vi "Close File.vi"(8 "error in (no error)":errorcluster, 11 "Parameter INI File in":refnum<class "Parameter INI File.lvclass">) -> (0 "error out":errorcluster, 3 "Parameter INI File out":refnum<class "Parameter INI File.lvclass">)   [LabVIEW 2016, in "CD Parameter Manager API.lvlib" / "Parameter INI File.lvclass"]
uses:
  Parameter INI File.lvclass
  <vilib>/Utility/config.llb/NI_LVConfig.lvlib
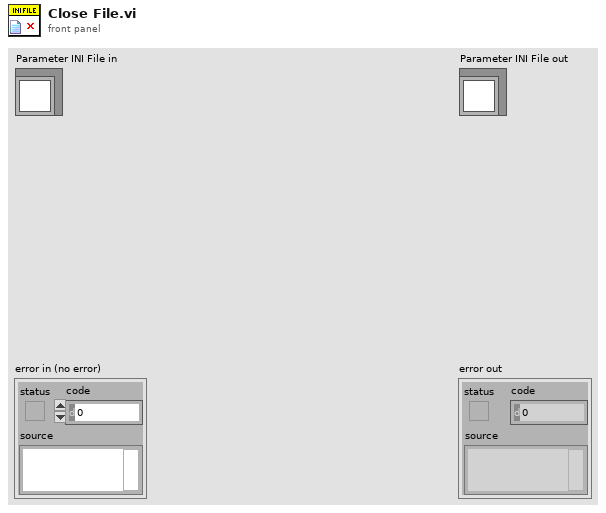
[diagram p1: front panel]
types:
  T1 = typedef "NI_LVConfig.lvlib/Config Data RefNum.ctl" = refnum<k1>
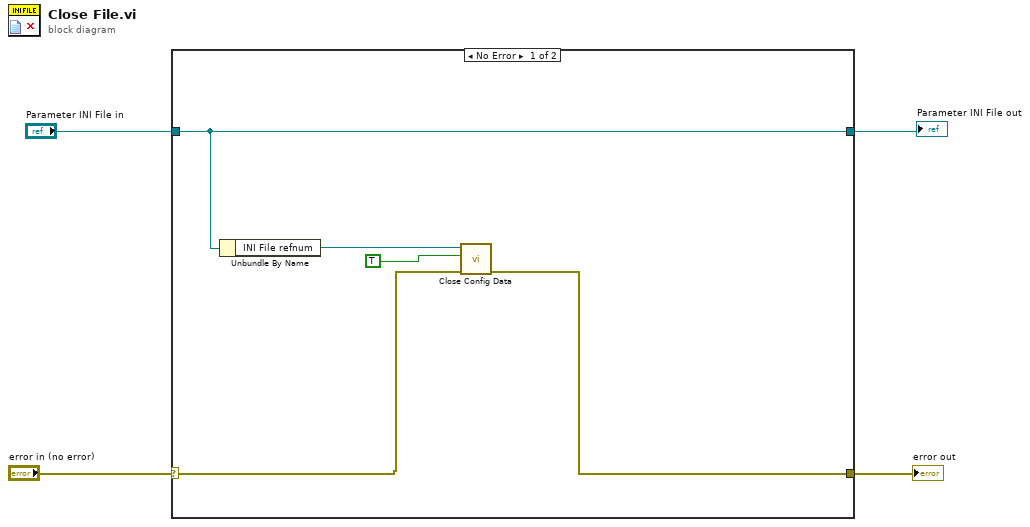
[diagram p0: block diagram]
diagram:
  n1 = case shown="No Error" "error in (no error)" {
    selector: "error in (no error)" -> [w7 w10]
    tunnel: [w9 w11] -> w2
    tunnel: "Parameter INI File in" -> [w9 w11]
    tunnel: [w6 w10] -> w1
    frame No Error {
      n2 = Unbundle By Name(w9) -> ("INI File refnum"=w8:T1)
      n3 = call <vilib>:"Close Config Data.vi"("error in (no error)"=w7, "write file if changed (T)"=TRUE, "refnum"=w8) -> ("error out"=w6:errorcluster)  [unwired: 7 in, 1 out]
    }
    frame Error {
    }
  }
  "error out" <- w1
  "Parameter INI File out" <- w2
